vi "Frequency Offset Estimation.vi"(8 "packet start valid":bool, 9 "packet start index":u16, 10 "auto correlation valid":bool, 11 "auto correlation":T1) -> (1 "output valid":bool, 2 "negated carrier frequency offset estimation":fxp<+/-,48,0>)   [LabVIEW 2020]
uses:
  <vilib>/rvi/FXPMathLib/FxpRectToPolar/subVIs/nifxpmath_RectToPolar_SimConfig.ctl
  <vilib>/rvi/Memory/Memory_Emulation/nirvimemoryEmulation.vi
  <vilib>/rvi/Memory/Memory_Emulation/nirvimemoryFastEmulation.vi
  <vilib>/rvi/DataTransferAndStorage/Container/Common/niFpgaContainerGetUniqueNameForEmu.vi
  <vilib>/rvi/Memory/Memory_Emulation/niFpgaMemoryEmulationCacheClearOnFirstRun.vi
  <vilib>/rvi/Memory/Memory_Emulation/nirvimemoryEmulationManagerCache_MakeExclusive.vi
  <vilib>/rvi/Memory/Memory_Emulation/niFpgaMemoryEmulationValidateCache.vi
  <vilib>/rvi/Memory/Memory_Emulation/nirvimemoryEmulationManagerCache_InsertValue.vi
  <vilib>/Utility/error.llb/Clear Errors.vi
  <vilib>/rvi/Memory/Memory_Emulation/nirvimemoryEmulationManagerCache_ReleaseExclusive.vi
  <vilib>/rvi/Memory/Memory_Emulation/nirvimemoryEmulationManagerCache_GetValue.vi
  <vilib>/rvi/Emulation/niFpgaEmulationIsFPGAContextNoSignature.vi
  <vilib>/rvi/Emulation/niFpgaSctlEmulationGetInTimedLoop.vi
  <vilib>/rvi/Memory/Memory_Emulation/nirvimemoryEmulationManagerCache_SetValue.vi
  <vilib>/rvi/Emulation/niFpgaSctlEmulationResourceMgr.vi
  <vilib>/rvi/FXPMathLib/FxpRectToPolar/simVIs/DllFxpRectToPolarTemp_sub.vi
  <vilib>/rvi/DataTransferAndStorage/Container/XNode/niFpgaContainer.xnode
  <vilib>/rvi/FXPMathLib/FxpMul/XNode/nifxpmath_Multiplier.xnode
  <vilib>/rvi/FXPMathLib/FxpRectToPolar/XNode/nifxpmath_RectToPolar.xnode
  <vilib>/rvi/FXPMathLib/sim/FxpSim.dll
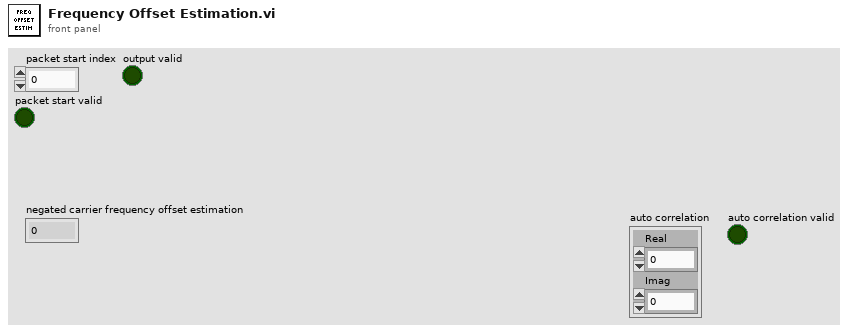
[diagram p1: front panel]
types:
  T1 = cluster{"Real":fxp<+/-,42,16>, "Imag":fxp<+/-,42,16>}
  T2 = cluster{"EIFS":u32, "ACK timeout":u32, "CTS timeout":u32, "aRxPHYStartDelay":u32, "Frame control field length":u16, "Duration/ID field length":u16, "aSlotTime":u32, "aSIFSTime":u32, "PIFS":u32, "DIFS":u32, "Address field length":u16, "Sequence control field length":u16, "QoS control field length":u16, "HT control field length":u16, "FCS field length":u16, "MPDU delimiter length":u16, "MPDU delimiter signature":u16, "Max MPDU buffer length":u16, "timestamp steps / mks":u32, "L-STF periods / L-STF":u8, "sample / L-STF period":u8, "T_SIGNAL":u16, "N_tail":u16, "N_service":u16, "N_ES":u16, "N_SS":u16, "m_STBC":u16, "T_VHTSIGB":u16, "T_VHTPREAMBLE":u16, "T_VHTSIGA":u16, "T_LSIG":u16, "T_LEGPREAMBLE":u16, "NOFDM_VHTSIGB":u16, "T_SYM":u16, "T_SYML":u16, "NOFDM_PREAMBLE":u16, "NOFDM_SIGNAL":u16, "T_PREAMBLE":u16, "NOFDM_LEGPREAMBLE":u16, "NOFDM_VHTPREAMBLE":u16, "NOFDM_VHTSIGA":u16, "NOFDM_LSIG":u16, "NOFDM_VHTPREAMBLE 2":u16, "NOFDM_LSIG 2":u16}
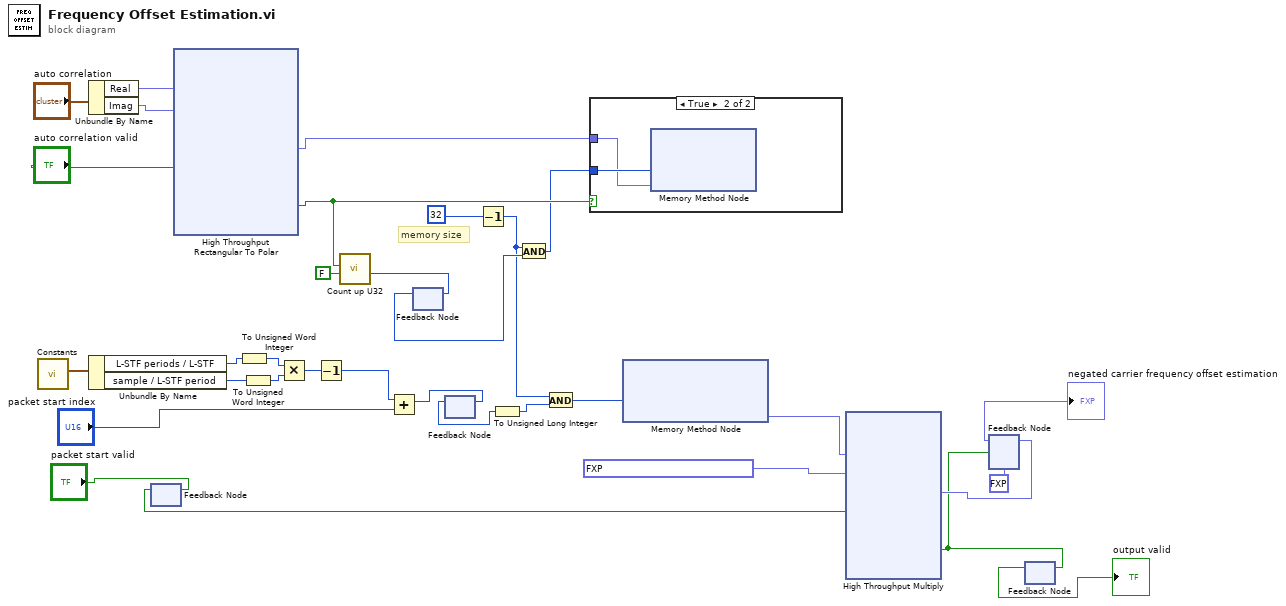
[diagram p0: block diagram]
diagram:
  # "memory size"
  n1 = call "Constants.vi"() -> ("output cluster"=w17:T2)  [unwired: 11 in]
  n2 = Unbundle By Name("auto correlation") -> ("Real"=w31:fxp<+/-,42,16>, "Imag"=w30:fxp<+/-,42,16>)
  n3 = Unbundle By Name(w17) -> ("L-STF periods / L-STF"=w22:u8, "sample / L-STF period"=w21:u8)
  n4 = feedback #1() -> (w9:bool)  [unwired: 1 in]
  n5 = feedback-in #1("packet start valid") -> ()
  n6 = xnode "High Throughput Rectangular To Polar"("x"=w31, "y"=w30, "input valid"="auto correlation valid") -> ("phase (pi)"=w23:fxp<+/-,24,2>, "output valid"=w28:bool)  [unwired: 1 in, 2 out]
  n7 = To Unsigned Word Integer(number=w22) -> (unsigned 16bit integer=w19:u16)
  n8 = To Unsigned Word Integer(number=w21) -> (unsigned 16bit integer=w20:u16)
  n9 = Multiply(x=w19, y=w20) -> (x*y=w18:u16)
  n10 = Decrement(x=w18) -> (x-1=w16:u16)
  n11 = call "Count up U32.vi"("reset"=FALSE, "increment"=w28) -> ("count out"=w25:u32)  [unwired: 9 in]
  n12 = Add(x=w16, y="packet start index") -> (x+y=w14:u16)
  n13 = feedback-in #2(w25) -> ()
  n14 = feedback #2() -> (w26:u32)  [unwired: 1 in]
  n15 = feedback #3() -> (w13:u16)  [unwired: 1 in]
  n16 = feedback-in #3(w14) -> ()
  n17 = Decrement(x=u32 32) -> (x-1=w11:u32)
  n18 = To Unsigned Long Integer(number=w13) -> (unsigned 32bit integer=w12:u32)
  n19 = And(x=w11, y=w26) -> (x .and. y?=w24:u32)
  n20 = And(x=w11, y=w12) -> (x .and. y?=w8:u32)
  n21 = case shown="True" w28 {
    tunnel: w24 -> [_ w35]
    tunnel: w23 -> [_ w34]
    frame False {
    }
    frame True {
      n22 = xnode ("Memory Method Node")("Address"=w35, "Data"=w34) -> ()  [unwired: 1 in, 1 out]
    }
  }
  n23 = xnode ("Memory Method Node")("Address"=w8) -> ("Data"=w7:fxp<+/-,24,2>)  [unwired: 1 in, 1 out]
  n24 = xnode ("High Throughput Multiply")("x"=w7, "y"=fxp<+/-,18,-8> -0.0015625059604644775, "input valid"=w9) -> ("x*y"=w6:fxp<+/-,48,0>, "output valid"=w3:bool)  [unwired: 1 in, 1 out]
  n25 = feedback #4(fxp<+/-,48,0> 0.0 ("x*y")) -> (→"negated carrier frequency offset estimation":fxp<+/-,48,0>)
  n26 = feedback-in #4(w6, w3) -> ()
  n27 = feedback #5() -> (→"output valid":bool)  [unwired: 1 in]
  n28 = feedback-in #5(w3) -> ()
